vi "ARC_Dynamic Load by Ref.vi"(6 "Auto Dispose Ref":bool, 8 "error in":errorcluster, 9 "CtrlValue":variant, 10 "CtrlName":string, 11 "Static vi reference in":refnum<vi>) -> (0 "错误输出":errorcluster caption="error out", 3 "Dynamic vi reference out":refnum<vi>)   [LabVIEW 2016]
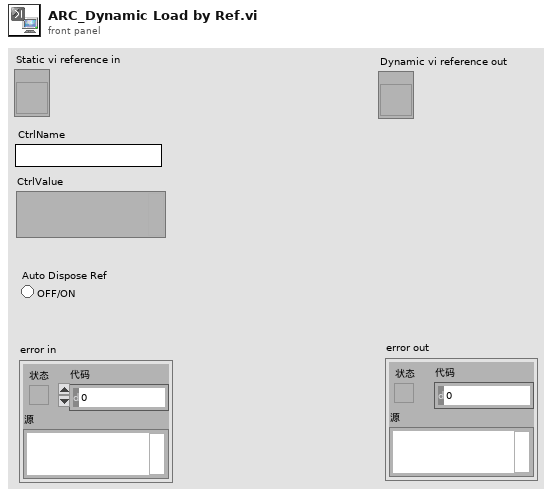
[diagram p1: front panel]
types:
  T1 = enum32{"Bad", "Idle", "Run top level", "Running"}
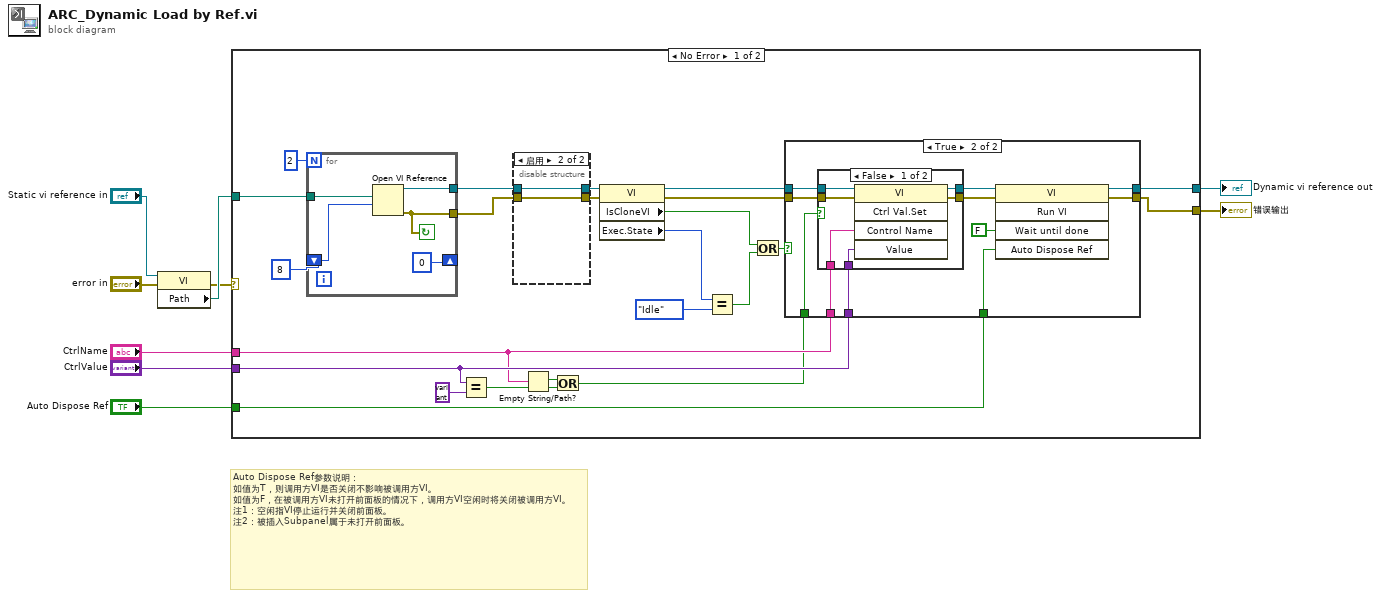
[diagram p0: block diagram]
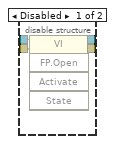
[diagram p2: hidden frame]
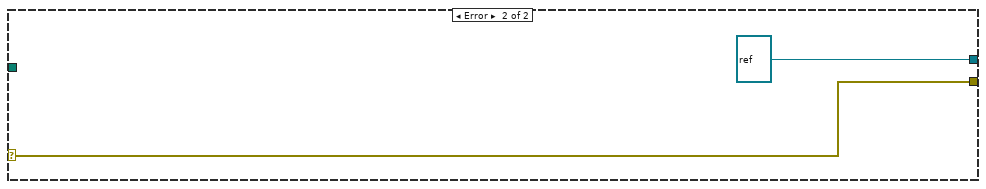
[diagram p5: hidden frame]
diagram:
  # "Auto Dispose Ref参数说明：\n如值为T，则调用方VI是否关闭不影响被调用方VI。\n如值为F，在被调用方VI未打开前面板的情况下，调用方VI空闲时将关闭被调用方VI。\n注1：空闲指VI停止运行并关闭前面板。\n注2：被插入Subpanel属于未打开前面板。"
  n1 = property class="VI"(reference="Static vi reference in", error in="error in") -> (error out=w1:errorcluster, "Path"=w3:path)  [unwired: 1 out]
  n2 = case shown="No Error" w1 {
    selector: w1 -> [_ w65]
    tunnel: [w23 refnum<vi> refnum ("vi reference")] -> w9
    tunnel: [w22 w65] -> w8
    tunnel: "Auto Dispose Ref" -> [w21 _]
    tunnel: "CtrlName" -> [w14 _]
    tunnel: "CtrlValue" -> [w16 _]
    tunnel: w3 -> [w10 _]
    frame No Error {
      n3 = for {
        N: 2 -> [_]
        tunnel: w10 -> [w43]
        shift-right: [0 ("选项")] -> _
        shift-left: 8 ("选项") -> [w42]
        tunnel: [w40] -> w18
        tunnel: [w39] -> w20
        stop <- w40 continue-if-true
        n4 = Open VI Reference(vi path=w43, options=w42) -> (vi reference=w39:refnum<vi>, error out=w40:errorcluster)  [unwired: 4 in]
      }
      n5 = Equal?(x=w16, y=variant) -> (x = y?=w12:bool)
      n6 = disable-structure shown="启用" {
        disable-tunnel: w20 -> [w36 w38]
        disable-tunnel: [w35 w38] -> w19
        disable-tunnel: w18 -> [w34 w37]
        disable-tunnel: [w33 w37] -> w17
        frame Disabled {
          n7 = invoke class="VI" method="FP.Open"(reference=w36, error in=w34) -> (reference out=w35:refnum<vi>, error out=w33:errorcluster)  [unwired: 3 in, 3 out]
        }
        frame Enabled {
        }
      }
      n8 = Empty String/Path?(string/path=w14) -> (empty?=w13:bool)
      n9 = Or(x=w13, y=w12) -> (x .or. y?=w11:bool)
      n10 = property class="VI"(reference=w19, error in=w17) -> (reference out=w32:refnum<vi>, error out=w31:errorcluster, "IsCloneVI"=w26:bool, "Exec.State"=w27:T1)
      n11 = Equal?(x=w27, y=T1."Idle") -> (x = y?=w25:bool)
      n12 = Or(x=w26, y=w25) -> (x .or. y?=w24:bool)
      n13 = case shown="True" w24 {
        tunnel: w32 -> [w45 w52]
        tunnel: [w45 w56] -> w23
        tunnel: w31 -> [w44 w50]
        tunnel: [w44 w55] -> w22
        tunnel: w21 -> [_ w53]
        tunnel: w14 -> [_ w48]
        tunnel: w16 -> [_ w47]
        tunnel: w11 -> [_ w46]
        frame False {
        }
        frame True {
          n14 = case shown="False" w46 {
            tunnel: w52 -> [w62 w64]
            tunnel: [w61 w64] -> w51
            tunnel: w50 -> [w60 w63]
            tunnel: [w59 w63] -> w49
            tunnel: w48 -> [w58 _]
            tunnel: w47 -> [w57 _]
            frame False {
              n15 = invoke class="VI" method="Ctrl Val.Set"(reference=w62, error in=w60, "Control Name"=w58, "Value"=w57) -> (reference out=w61:refnum<vi>, error out=w59:errorcluster)  [unwired: 1 in, 3 out]
            }
            frame True {
            }
          }
          n16 = invoke class="VI" method="Run VI"(reference=w51, error in=w49, "Wait until done"=FALSE ("结束前等待"), "Auto Dispose Ref"=w53) -> (reference out=w56:refnum<vi>, error out=w55:errorcluster)  [unwired: 1 in, 3 out]
        }
      }
    }
    frame Error {
    }
  }
  "Dynamic vi reference out" <- w9
  "错误输出" <- w8
